vi "Construct CellFormat.vi"(8 "error in":errorcluster, 11 "Formats":T1={"NumberFormatId"=164, "FontId"=0, "FillId"=0, "BorderId"=0, "FormatId"=0, "ApplyNumberFormat"=TRUE}) -> (0 "error out":errorcluster, 3 "CellFormat":refnum<k24>)   [LabVIEW 2021, in "Open Xml.lvlib"]
uses:
  Open Xml.lvlib
  D:/git/Open-Xml-LabVIEW/dll/DocumentFormat.OpenXml.Framework.dll
  dll/DocumentFormat.OpenXml.Framework.dll
  D:/git/Open-Xml-LabVIEW/dll/DocumentFormat.OpenXml.dll
  dll/DocumentFormat.OpenXml.dll
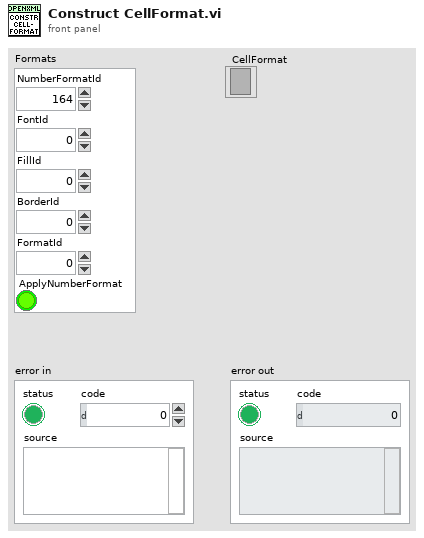
[diagram p1: front panel]
types:
  T1 = cluster{"NumberFormatId":u32, "FontId":u32, "FillId":u32, "BorderId":u32, "FormatId":u32, "ApplyNumberFormat":bool}
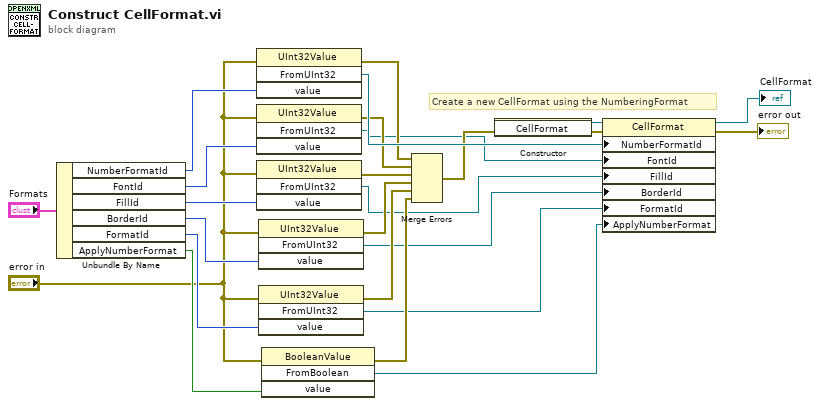
[diagram p0: block diagram]
diagram:
  # "Create a new CellFormat using the NumberingFormat"
  n1 = Unbundle By Name("Formats") -> ("NumberFormatId"=w20:u32, "FontId"=w19:u32, "FillId"=w18:u32, "BorderId"=w17:u32, "FormatId"=w16:u32, "ApplyNumberFormat"=w15:bool)
  n2 = invoke class="UInt32Value" method="FromUInt32"(error in="error in", "value"=w20) -> (error out=w13:errorcluster, "FromUInt32"=w14:refnum<k24>)  [unwired: 2 in, 2 out]
  n3 = invoke class="UInt32Value" method="FromUInt32"(error in="error in", "value"=w19) -> (error out=w12:errorcluster, "FromUInt32"=w6:refnum<k24>)  [unwired: 2 in, 2 out]
  n4 = invoke class="UInt32Value" method="FromUInt32"(error in="error in", "value"=w18) -> (error out=w11:errorcluster, "FromUInt32"=w5:refnum<k24>)  [unwired: 2 in, 2 out]
  n5 = invoke class="UInt32Value" method="FromUInt32"(error in="error in", "value"=w17) -> (error out=w10:errorcluster, "FromUInt32"=w4:refnum<k24>)  [unwired: 2 in, 2 out]
  n6 = invoke class="UInt32Value" method="FromUInt32"(error in="error in", "value"=w16) -> (error out=w9:errorcluster, "FromUInt32"=w2:refnum<k24>)  [unwired: 2 in, 2 out]
  n7 = invoke class="BooleanValue" method="FromBoolean"(error in="error in", "value"=w15) -> (error out=w8:errorcluster, "FromBoolean"=w3:refnum<k24>)  [unwired: 2 in, 2 out]
  n8 = Merge Errors(w13, w12, w11, w10, w9, w8) -> (w7:errorcluster)
  n9 = constructor class="CellFormat"(error in=w7) -> (reference out=w23:refnum<k24>, error out=w24:errorcluster)  [unwired: 2 in, 1 out]
  n10 = property class="CellFormat"(reference=w23, error in=w24, "NumberFormatId"=w14, "FontId"=w6, "FillId"=w5, "BorderId"=w4, "FormatId"=w2, "ApplyNumberFormat"=w3) -> (reference out=→"CellFormat":refnum<k24>, error out=→"error out":errorcluster)
